vi "MasterBoundsToRect.vi"(8 "error in":errorcluster, 11 "Owner Bounds":T1) -> (0 "error out":errorcluster, 3 "JSON":string)   [LabVIEW 2017]
doc: "Converts Master Rect into JSON format with x, y, width and height"
uses:
  <vilib>/Utility/miscctls.llb/LVRectTypeDef.ctl
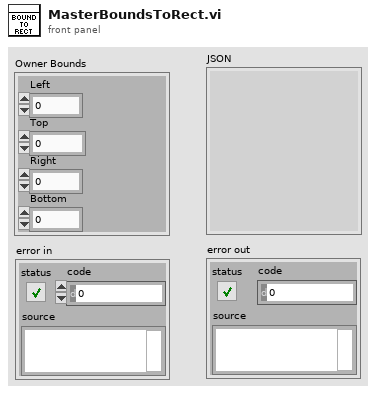
[diagram p1: front panel]
types:
  T1 = typedef "LVRectTypeDef.ctl" = cluster{"Left":i16, "Top":i16, "Right":i16, "Bottom":i16}
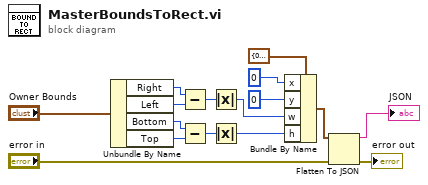
[diagram p0: block diagram]
diagram:
  n1 = Unbundle By Name("Owner Bounds") -> ("Right"=w15:i16, "Left"=w10:i16, "Bottom"=w14:i16, "Top"=w9:i16)
  n2 = Subtract(x=w15, y=w10) -> (x-y=w11:i16)
  n3 = Subtract(x=w14, y=w9) -> (x-y=w13:i16)
  n4 = Absolute Value(x=w11) -> (abs(x)=w4:i16)
  n5 = Absolute Value(x=w13) -> (abs(x)=w3:i16)
  n6 = Bundle By Name(cluster=cluster{"x":i32, "y":i32, "w":i32, "h":i32} {"x"=0, "y"=0, "w"=0, "h"=0} ("Rect 2"), "x"=0, "y"=0, "w"=w4, "h"=w3) -> (w8:cluster{"x":i32, "y":i32, "w":i32, "h":i32})
  n7 = Flatten To JSON(anything=w8, error in (no error)="error in") -> (JSON string=→"JSON":string, 11:→"error out":errorcluster)  [unwired: 1 in]
